vi "cool_amp.vi"() -> ()   [LabVIEW 2011]
uses:
  <vilib>/LabVIEW Interface for Arduino/Type Defs/Digital Pin.ctl
  <vilib>/LabVIEW Interface for Arduino/Type Defs/Pin Mode.ctl
  <vilib>/LabVIEW Interface for Arduino/LabVIEW Interface for Arduino.lvlib
  <vilib>/Analysis/NI_AALBase.lvlib
panel:
  in  "Tab Control":T1(tab)
  in  "save & stop":bool
  out "System Status":bool
  in  "Clear History":bool
  in  "average time":i32=4 min=0 step=1
  in  "Quit Program":bool
  in  "Start":bool
  in  "Stop":bool
  out "T3 Over Limit":bool caption="T3 over limit"
  out "T2 Over Limit":bool caption="T2 over limit"
  out "T1 Over Limit":bool caption="T1 over limit"
  out "Flow Graph":cluster{dbl[], dbl[]}(graph)
  out "flow rate":dbl=4.0 format="%3.1f"
  out "mean flow":dbl=4.0 format="%5.1f"
  out "total cost ($)":dbl=4.0 format="%05.2f"
  out "total flow (L)":dbl=4.0 format="%6.1g"
  out "current flow rate":dbl(slide)=4.0 scale=0.0..20.0
  out "Temp Graph":cluster{dbl[], dbl[]}[](graph)
  out "delta T3":dbl=4.0 format="%6.1g"
  out "delta T2":dbl=4.0 format="%6.1g"
  out "delta T1":dbl=4.0 format="%6.1g"
  out "T3 average":dbl=4.0 format="%6.1f"
  out "T2 average":dbl=4.0 format="%6.1f"
  out "T1 average":dbl=4.0 format="%6.1f"
  out "T3":dbl(slide) scale=-40.0..40.0 scale format="%#_3f"
  out "T2":dbl(slide) scale=-40.0..40.0 scale format="%#_3f"
  out "T1":dbl(slide) scale=-40.0..40.0
  out "T1 numeric":dbl=4.0 format="%6.1f"
  out "T2 numeric":dbl=4.0 format="%6.1f"
  out "T3 numeric":dbl=4.0 format="%6.1f"
  out "T1 max":dbl=4.0 format="%0#3_3g"
  out "T1 min":dbl=4.0 format="%0#3_3g"
  out "T1 average":dbl=4.0 format="%0#3_3g"
  out "T2 max":dbl=4.0 format="%0#3_3g"
  out "T2 min":dbl=4.0 format="%0#3_3g"
  out "T2 average":dbl=4.0 format="%0#3_3g"
  out "T3 max":dbl=4.0 format="%0#3_3g"
  out "T3 min":dbl=4.0 format="%0#3_3g"
  out "T3 average":dbl=4.0 format="%0#3_3g"
  out "max flow":dbl=4.0 format="%#3.1p"
  out "min flow":dbl=4.0 format="%5.1f"
  out "average flow":dbl=4.0 format="%#5.1f"
  out "Arduino \nConnection":bool
  in  "Arduino Serial Port":refnum<visa-resource-name>="ArduinoUno"
  in  "Flow Low Limit":dbl=3.0 min=0.0
  in  "T3 High Limit":dbl=30.0
  in  "T2 High Limit":dbl=30.0
  in  "T1 High Limit":dbl=-20.0
  in  "LED Pin":T2=enum."Pin13"
  out "Total Count":u32=4
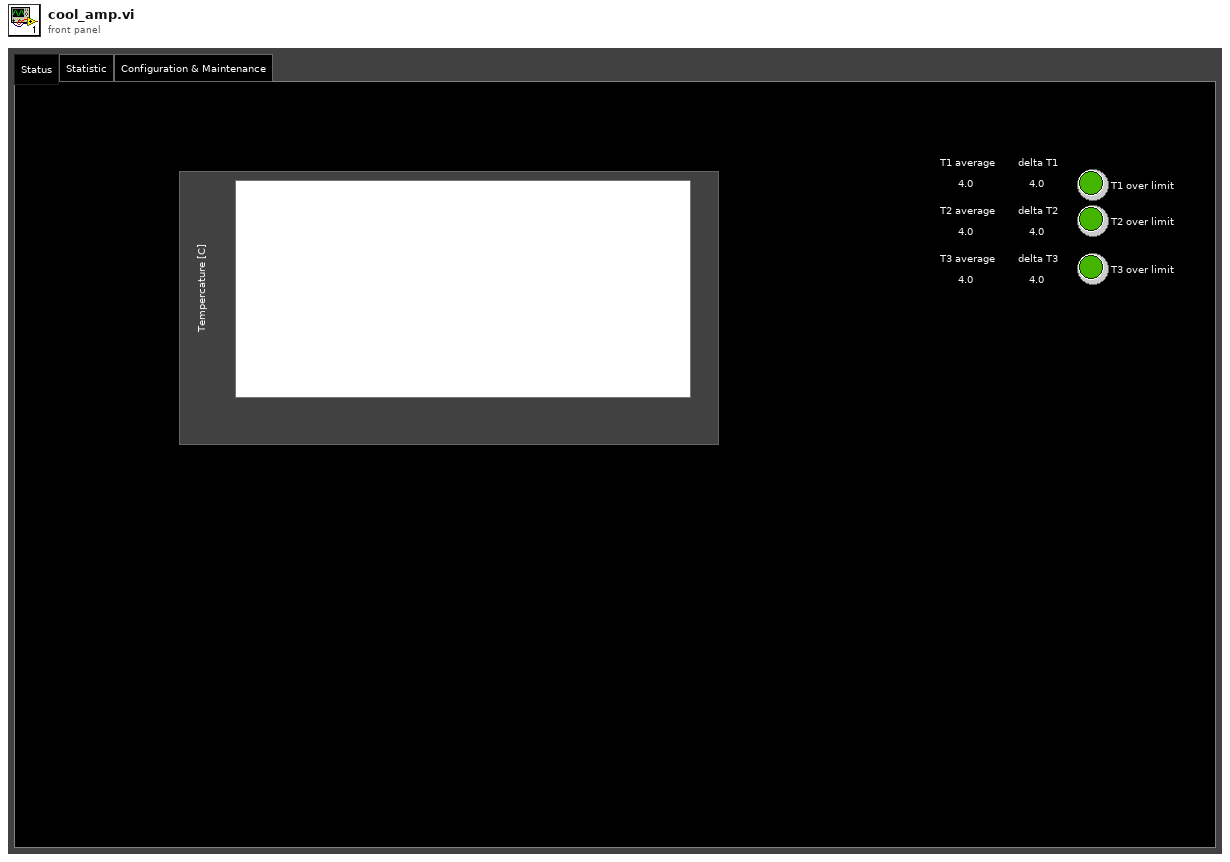
[diagram p1: front panel]
types:
  T1 = enum32{"Status", "Statistic", "Configuration & Maintenance"}
  T2 = typedef "LabVIEW Interface for Arduino.lvlib/Digital Pin.ctl" = enum8{"Pin0", "Pin1", "Pin2", "Pin3", "Pin4", "Pin5", "Pin6", "Pin7", "Pin8", "Pin9", "Pin10", "Pin11", "Pin12", "Pin13"}
  T3 = enum8{"Enabled", "Disabled", "Disabled and Grayed Out"}
  T4 = enum8{"setArduinoMode", "flushSerial", "setPinMode", "digitalWritePin", "digitalWritePort", "tone", "digitalReadPin", "digitalReadPort", "analogReadPin", "analogReadPort", "pwmWritePin", "pwmWritePort", "sevenSegment_Configure", "sevenSegment_Write", "I2C Init", "I2C Write", "I2C Read", "SPI Init", "SPI Set Bit Order", "SPI Set Clock Divider", "SPI Set Data Mode", "SPI Send / Receive", "SPI Close", "Servo Set Num Servos", "Servo Config Servo", "Servo Write Angle", "Servo Read Angle", "Servo Write Pulse Width", "Servo Read Pulse Width", "Servo Detach", "LCD Init", "LCD Set Size", "LCD Set Cursor Mode", "LCD Clear", "LCD Set Cursor Position", "LCD Print", "LCD Display Power", "LCD Scroll Display", "LCD Autoscroll", "LCD Print Direction", "LCD Create Custom Char", "LCD Print Custom Char", "contAcqOn", "contAcqOff", "getFirmwareVersion", "FiniteSampleStart", "readFlowmeter_freq", "readFlowmeter_totalcount"}
  T5 = typedef "LabVIEW Interface for Arduino.lvlib/Pin Mode.ctl" = enum8{"Input", "Output"}
  T6 = typedef "LabVIEW Interface for Arduino.lvlib/Arduino Resource.ctl" = cluster{"VISA resource":refnum<visa-resource-name>, "Board Type":T7, "Connection Type":enum8{"USB / Serial"}, "Bytes Per Packet (15)":u8}
  T7 = typedef "LabVIEW Interface for Arduino.lvlib/Board Type.ctl" = enum16{"Uno", "Dimuelanove w/Atmega 328", "Mega 2560"}
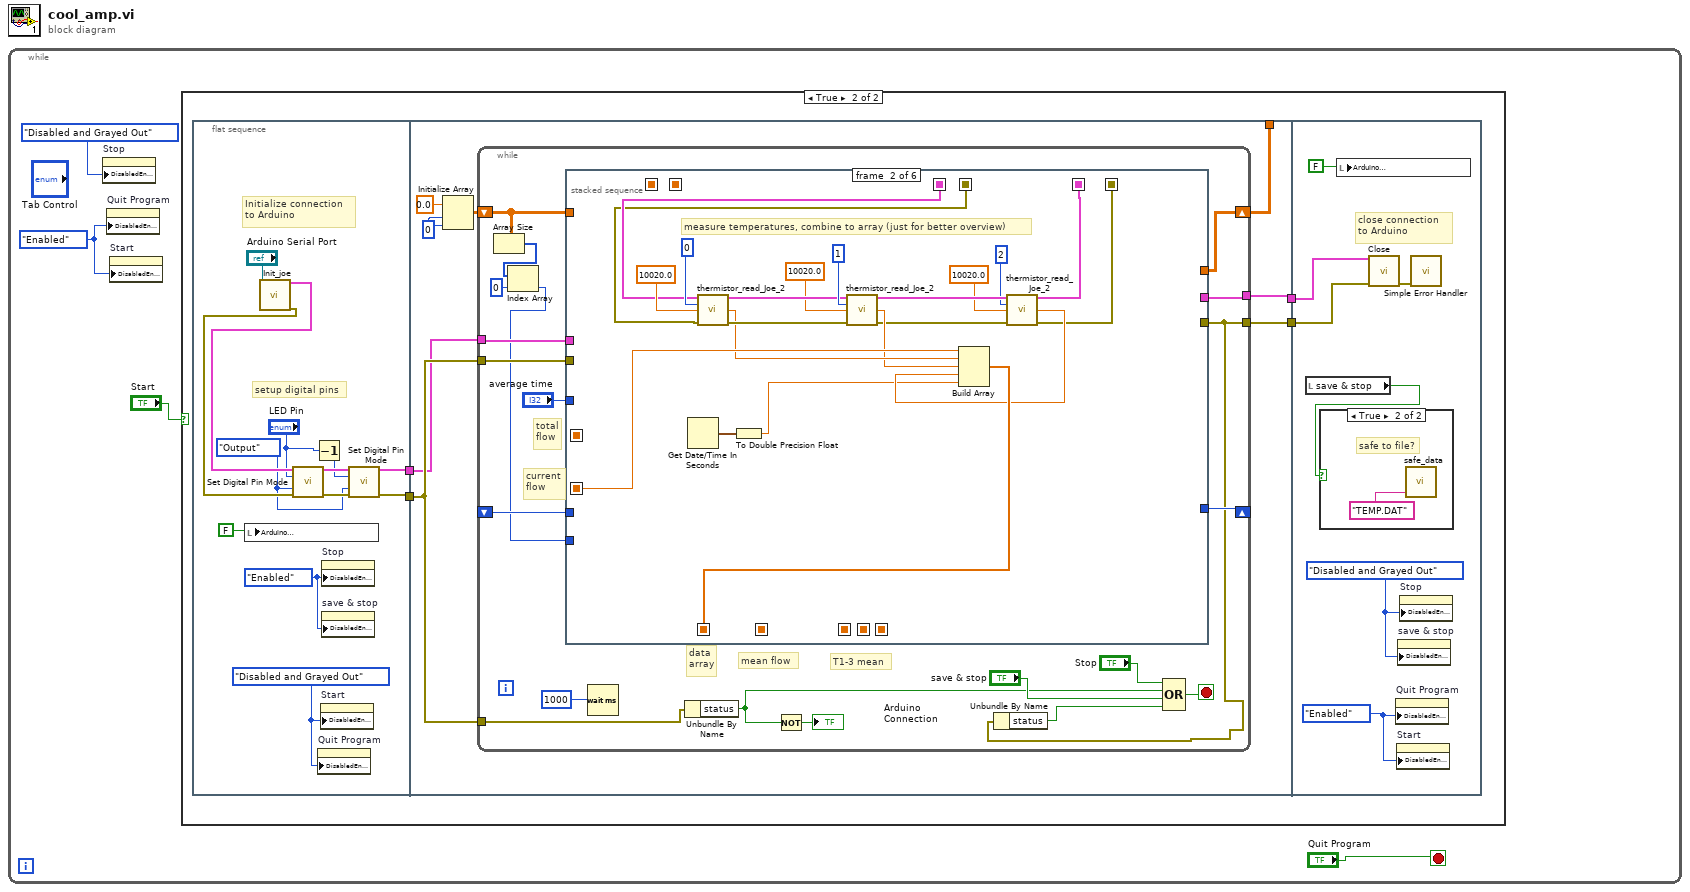
[diagram p0: block diagram]
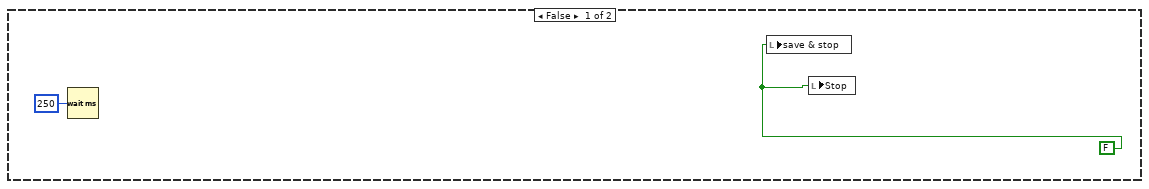
[diagram p2: hidden frame]
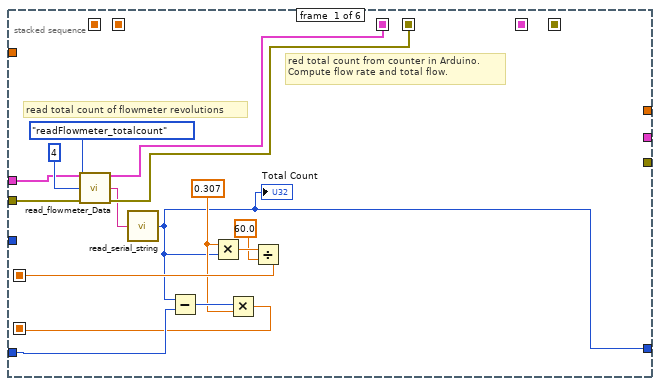
[diagram p3: hidden frame]
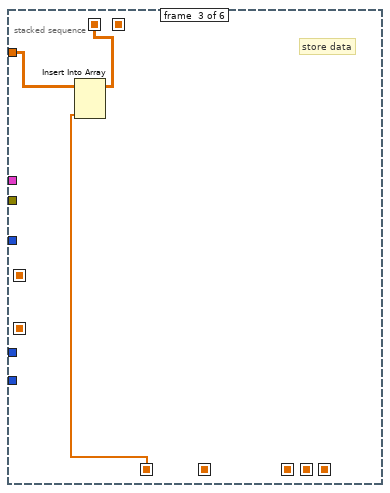
[diagram p4: hidden frame]
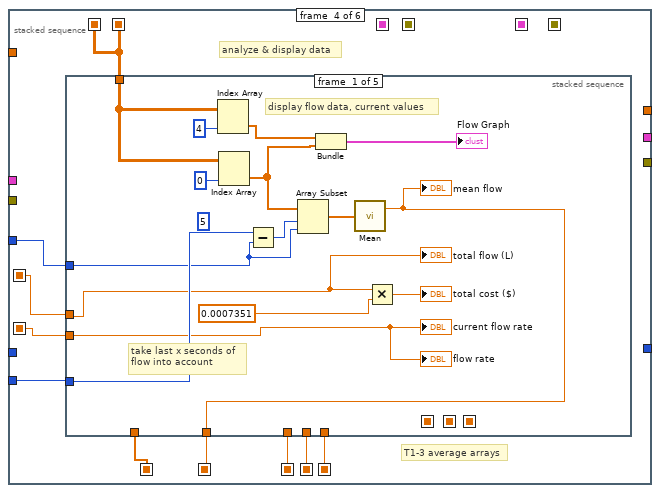
[diagram p5: hidden frame]
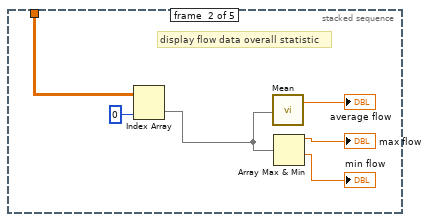
[diagram p6: hidden frame]
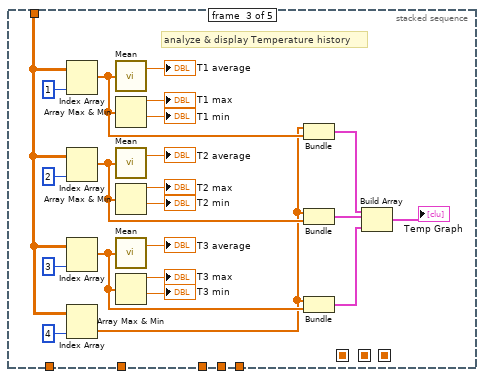
[diagram p7: hidden frame]
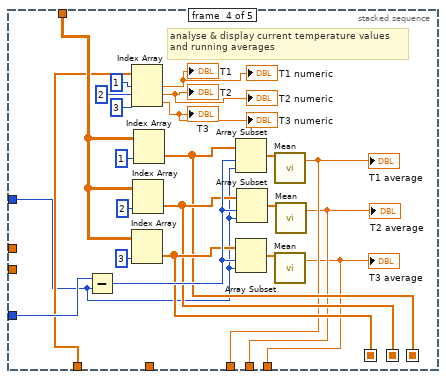
[diagram p8: hidden frame]
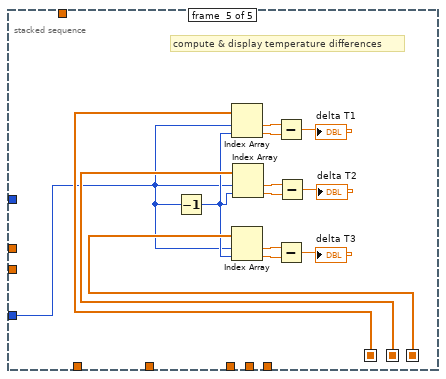
[diagram p9: hidden frame]
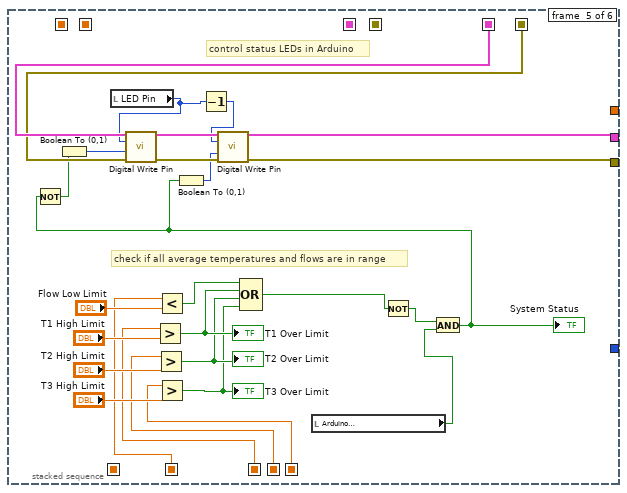
[diagram p10: hidden frame]
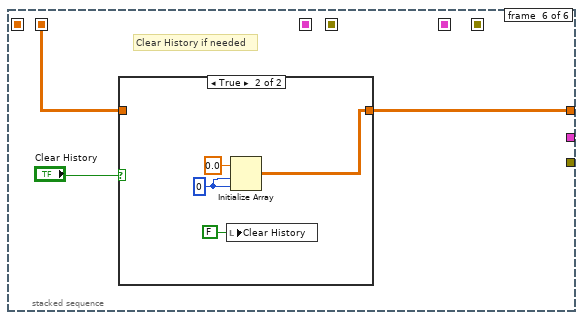
[diagram p11: hidden frame]
diagram:
  n1 = while {
    stop <- "Quit Program" stop-if-true
    w2 = T3."Enabled" ("Disabled")
    n2 = property on="Stop" class="Bool (strict)"("DisabledEnum"=T3."Disabled and Grayed Out" ("Disabled")) -> ()  [unwired: 2 in, 2 out]
    n3 = property on="Quit Program" class="Bool"("DisabledEnum"=w2) -> ()  [unwired: 2 in, 2 out]
    n4 = property on="Start" class="Bool"("DisabledEnum"=w2) -> ()  [unwired: 2 in, 2 out]
    n5 = case shown="True" "Start" {
      frame False {
        w5 = FALSE
        n6 = Wait (ms)(milliseconds to wait=u32 250) -> ()  [unwired: 1 out]
        n7 = local write "save & stop"(w5) -> ()
        n8 = local write "Stop"(w5) -> ()
      }
      frame True {
        n9 = flat-sequence {
          tunnel: [w16] -> w10
          tunnel: [w18] -> w9
          tunnel: w10 -> [w29]
          tunnel: w9 -> [w31]
          tunnel: [w28] -> w8
          tunnel: [w27] -> w7
          tunnel: [w24] -> _
          tunnel: w8 -> [w219]
          tunnel: w7 -> [w220]
          frame #0 {
            w13 = Pin_Mode."Output" ("Pin Mode (Input)")
            w12 = T3."Enabled" ("Disabled")
            w11 = T3."Disabled and Grayed Out" ("Disabled")
            # "setup digital pins"
            # "Initialize connection \nto Arduino"
            n10 = local write "Arduino \nConnection"(FALSE) -> ()
            n11 = call "Init_joe.vi"("VISA resource"="Arduino Serial Port") -> ("Arduino Resource"=w19:T6, "error out"=w21:errorcluster)  [unwired: 17 in]
            n12 = call <vilib>:"Set Digital Pin Mode.vi"("Arduino Resource"=w19, "Digital I/O Pin"="LED Pin", "Pin Mode (Input)"=w13, "error in"=w21) -> ("Arduino Resource"=w17:T6, "error out"=w20:errorcluster)  [unwired: 10 in]
            n13 = Decrement(x="LED Pin") -> (x-1=w14:T2)
            n14 = property on="Quit Program" class="Bool"("DisabledEnum"=w11) -> ()  [unwired: 2 in, 2 out]
            n15 = property on="Start" class="Bool"("DisabledEnum"=w11) -> ()  [unwired: 2 in, 2 out]
            n16 = property on="Stop" class="Bool (strict)"("DisabledEnum"=w12) -> ()  [unwired: 2 in, 2 out]
            n17 = property on="save & stop" class="Bool (strict)"("DisabledEnum"=w12) -> ()  [unwired: 2 in, 2 out]
            n18 = call <vilib>:"Set Digital Pin Mode.vi"("Arduino Resource"=w17, "Digital I/O Pin"=w14, "Pin Mode (Input)"=w13, "error in"=w20) -> ("Arduino Resource"=w16:T6, "error out"=w18:errorcluster)  [unwired: 10 in]
          }
          frame #1 {
            w30 = 0 ("dimension size")
            n19 = Initialize Array(0.0 ("element"), w30, w30) -> (w25:dbl[][])
            n20 = while {
              tunnel: w29 -> [w47]
              tunnel: w31 -> [w46]
              shift-right: [w43] -> w24
              shift-left: w25 -> [w42]
              tunnel: w31 -> [w49]
              tunnel: [w48] -> w28
              tunnel: [w34] -> w27
              shift-right: [w44] -> _
              shift-left: _ -> [w45]
              stop <- w37 stop-if-true
              # "mean flow"
              # "T1-3 mean"
              # "total\nflow"
              # "data\narray"
              # "current\nflow"
              n21 = Array Size(array=w42) -> (size(s)=w41:i32[])
              n22 = Index Array(array=w41, index=0) -> (element=w33:i32)
              n23 = stacked-sequence {
                seq-local: [w52 _ _ _ _ _] -> [_ w81 _ _ _ _]
                seq-local: [w58 _ _ _ _ _] -> [_ w80 _ _ _ _]
                seq-local: [w54 _ _ _ _ _] -> [_ w79 _ w99 _ _]
                seq-local: [_ w77 _ _ _ _] -> [_ _ w88 w93 _ _]
                seq-local: [w62 _ _ _ _ _] -> [_ _ _ w98 _ _]
                seq-local: [_ w70 _ _ _ _] -> [_ _ _ _ w190 _]
                seq-local: [_ w69 _ _ _ _] -> [_ _ _ _ w189 _]
                seq-local: [_ _ _ w91 _ _] -> [_ _ _ _ _ w210]
                seq-local: [_ _ _ w97 _ _] -> [_ _ _ _ w199 _]
                seq-local: [_ _ _ w96 _ _] -> [_ _ _ _ w198 _]
                seq-local: [_ _ _ w95 _ _] -> [_ _ _ _ w197 _]
                seq-local: [_ _ _ w94 _ _] -> [_ _ _ _ w195 _]
                seq-local: [_ _ w89 _ _ _] -> [_ _ _ w91 _ _]
                tunnel: [_ _ _ _ w188 _] -> w48
                tunnel: [_ _ _ _ w186 _] -> w34
                tunnel: w47 -> [w61 _ _ _ _ _]
                tunnel: w46 -> [w60 _ _ _ _ _]
                tunnel: w42 -> [_ _ w90 _ _ _]
                tunnel: w33 -> [_ _ _ w100 _ _]
                tunnel: w45 -> [w56 _ _ _ _ _]
                tunnel: [w53 _ _ _ _ _] -> w44
                tunnel: [_ _ _ _ _ w209] -> w43
                tunnel: "average time" -> [_ _ _ w92 _ _]
                frame #0 {
                  w55 = 0.307
                  # "read total count of flowmeter revolutions"
                  # "red total count from counter in Arduino. \nCompute flow rate and total flow."
                  n24 = call "read_flowmeter_Data.vi"("Arduino Resource"=w61, "Command"=T4."readFlowmeter_totalcount", "Bytes To Read (0)"=u8 4, "error in"=w60) -> ("Arduino Resource"=w52:T6, "Read Buffer"=w57:string, "error out"=w58:errorcluster)  [unwired: 9 in]
                  n25 = call "read_serial_string.vi"("serial read Buffer"=w57) -> ("unsigned long"=w53:u32)  [unwired: 4 in]
                  "Total Count" <- w53
                  n26 = Subtract(x=w53, y=w56) -> (x-y=w59:u32)
                  n27 = Multiply(x=w55, y=w53) -> (x*y=w64:dbl)
                  n28 = Multiply(x=w59, y=w55) -> (x*y=w54:dbl)
                  n29 = Divide(x=w64, y=60.0) -> (x/y=w62:dbl)
                }
                frame #1 {
                  # "measure temperatures, combine to array (just for better overview)"
                  n30 = Get Date/Time In Seconds() -> (seconds since 1Jan1904=w68:timestamp)
                  n31 = call "thermistor_read_Joe_2.vi"("Arduino Resource"=w81, "Thermistor AI Pin (0)"=u8 0 ("T1 Pin"), "Paired Resistance (10K Ohms)"=10020.0, "error in"=w80) -> ("Arduino Resource"=w84:T6, "Temperature"=w78:dbl, "error out"=w83:errorcluster)  [unwired: 9 in]
                  n32 = To Double Precision Float(number=w68) -> (double precision float=w67:dbl)
                  n33 = call "thermistor_read_Joe_2.vi"("Arduino Resource"=w84, "Thermistor AI Pin (0)"=u8 1 ("T2 Pin"), "Paired Resistance (10K Ohms)"=10020.0, "error in"=w83) -> ("Arduino Resource"=w75:T6, "Temperature"=w76:dbl, "error out"=w74:errorcluster)  [unwired: 9 in]
                  n34 = call "thermistor_read_Joe_2.vi"("Arduino Resource"=w75, "Thermistor AI Pin (0)"=u8 2 ("T2 Pin"), "Paired Resistance (10K Ohms)"=10020.0, "error in"=w74) -> ("Arduino Resource"=w70:T6, "Temperature"=w71:dbl, "error out"=w69:errorcluster)  [unwired: 9 in]
                  n35 = Build Array(w79, w78, w76, w71, w67) -> (w77:dbl[])
                }
                frame #2 {
                  # "store data"
                  n36 = Insert Into Array(array=w90, new element=w88) -> (w89:dbl[][])  [unwired: 2 in]
                }
                frame #3 {
                  # "T1-3 average arrays"
                  # "analyze & display data"
                  n37 = stacked-sequence {
                    seq-local: [_ _ _ w151 _] -> [_ _ _ _ w180]
                    seq-local: [_ _ _ w150 _] -> [_ _ _ _ w170]
                    seq-local: [_ _ _ w148 _] -> [_ _ _ _ w169]
                    tunnel: w91 -> [w102 w117 w124 w159 _]
                    tunnel: w100 -> [w113 _ _ w162 w167]
                    tunnel: w99 -> [w108 _ _ _ _]
                    tunnel: w98 -> [w109 _ _ _ _]
                    tunnel: w93 -> [_ _ _ w149 _]
                    tunnel: [_ _ _ w147 _] -> w97
                    tunnel: [_ _ _ w146 _] -> w96
                    tunnel: [_ _ _ w145 _] -> w95
                    tunnel: [w105 _ _ _ _] -> w94
                    tunnel: w92 -> [w104 _ _ w144 _]
                    frame #0 {
                      (unwired) 5 ("disabled index (col)")
                      # "display flow data, current values"
                      # "take last x seconds of \nflow into account"
                      n38 = Index Array(array=w102, index (col)=4 ("disabled index (col)")) -> (element=w103:dbl[])  [unwired: 1 in]
                      n39 = Index Array(array=w102, index (col)=0 ("disabled index (col)")) -> (element=w106:dbl[])  [unwired: 1 in]
                      n40 = Subtract(x=w113, y=w104) -> (x-y=w114:i32)
                      n41 = Array Subset(array=w106, index=w114, length=w104) -> (w112:dbl[])
                      n42 = Bundle(w103, w106) -> (→"Flow Graph":cluster{dbl[], dbl[]})  [unwired: 1 in]
                      n43 = call <vilib>:"Mean.vi"("X"=w112) -> ("mean"=w105:dbl)  [unwired: 1 out]
                      "mean flow" <- w105
                      n44 = Multiply(x=w109, y=0.0007351) -> (x*y=→"total cost ($)":dbl)
                      "current flow rate" <- w108
                      "total flow (L)" <- w109
                      "flow rate" <- w108
                    }
                    frame #1 {
                      # "display flow data overall statistic"
                      n45 = Index Array(array=w117, index (col)=0 ("disabled index (col)")) -> (element=w116:dbl[])  [unwired: 1 in]
                      n46 = call <vilib>:"Mean.vi"("X"=w116) -> ("mean"=→"average flow":dbl)  [unwired: 1 out]
                      n47 = Array Max & Min(array=w116) -> (max value=→"max flow":dbl, min value=→"min flow":dbl)  [unwired: 2 out]
                    }
                    frame #2 {
                      # "analyze & display Temperature history"
                      n48 = Index Array(array=w124, index (col)=1 ("disabled index (col)")) -> (element=w128:dbl[])  [unwired: 1 in]
                      n49 = Index Array(array=w124, index (col)=2 ("disabled index (col)")) -> (element=w127:dbl[])  [unwired: 1 in]
                      n50 = Index Array(array=w124, index (col)=3 ("disabled index (col)")) -> (element=w126:dbl[])  [unwired: 1 in]
                      n51 = Index Array(array=w124, index (col)=4 ("disabled index (col)")) -> (element=w123:dbl[])  [unwired: 1 in]
                      n52 = call <vilib>:"Mean.vi"("X"=w128) -> ("mean"=→"T1 average":dbl)  [unwired: 1 out]
                      n53 = Array Max & Min(array=w128) -> (max value=→"T1 max":dbl, min value=→"T1 min":dbl)  [unwired: 2 out]
                      n54 = call <vilib>:"Mean.vi"("X"=w127) -> ("mean"=→"T2 average":dbl)  [unwired: 1 out]
                      n55 = Array Max & Min(array=w127) -> (max value=→"T2 max":dbl, min value=→"T2 min":dbl)  [unwired: 2 out]
                      n56 = call <vilib>:"Mean.vi"("X"=w126) -> ("mean"=→"T3 average":dbl)  [unwired: 1 out]
                      n57 = Array Max & Min(array=w126) -> (max value=→"T3 max":dbl, min value=→"T3 min":dbl)  [unwired: 2 out]
                      n58 = Bundle(w123, w128) -> (w130:cluster{dbl[], dbl[]})  [unwired: 1 in]
                      n59 = Bundle(w123, w127) -> (w131:cluster{dbl[], dbl[]})  [unwired: 1 in]
                      n60 = Bundle(w123, w126) -> (w129:cluster{dbl[], dbl[]})  [unwired: 1 in]
                      n61 = Build Array(w130, w131, w129) -> (→"Temp Graph":cluster{dbl[], dbl[]}[])
                    }
                    frame #3 {
                      # "analyse & display current temperature values\nand running averages"
                      n62 = Subtract(x=w162, y=w144) -> (x-y=w158:i32)
                      n63 = Index Array(array=w149, index #1=1, index #2=2, index #3=3) -> (element #1=→"T1" →"T1 numeric":dbl, element #2=→"T2" →"T2 numeric":dbl, element #3=→"T3" →"T3 numeric":dbl)
                      n64 = Index Array(array=w159, index (col)=3 ("disabled index (col)")) -> (element=w151:dbl[])  [unwired: 1 in]
                      n65 = Index Array(array=w159, index (col)=2 ("disabled index (col)")) -> (element=w150:dbl[])  [unwired: 1 in]
                      n66 = Index Array(array=w159, index (col)=1 ("disabled index (col)")) -> (element=w148:dbl[])  [unwired: 1 in]
                      n67 = Array Subset(array=w148, index=w158, length=w144) -> (w153:dbl[])
                      n68 = Array Subset(array=w151, index=w158, length=w144) -> (w154:dbl[])
                      n69 = Array Subset(array=w150, index=w158, length=w144) -> (w152:dbl[])
                      n70 = call <vilib>:"Mean.vi"("X"=w153) -> ("mean"=w147:dbl)  [unwired: 1 out]
                      "T1 average" <- w147
                      n71 = call <vilib>:"Mean.vi"("X"=w154) -> ("mean"=w145:dbl)  [unwired: 1 out]
                      "T3 average" <- w145
                      n72 = call <vilib>:"Mean.vi"("X"=w152) -> ("mean"=w146:dbl)  [unwired: 1 out]
                      "T2 average" <- w146
                    }
                    frame #4 {
                      # "compute & display temperature differences"
                      n73 = Decrement(x=w167) -> (x-1=w168:i32)
                      n74 = Index Array(array=w180, index #1=w167, index #2=w168) -> (element #1=w179:dbl, element #2=w178:dbl)
                      n75 = Index Array(array=w169, index #1=w167, index #2=w168) -> (element #1=w173:dbl, element #2=w172:dbl)
                      n76 = Index Array(array=w170, index #1=w167, index #2=w168) -> (element #1=w176:dbl, element #2=w175:dbl)
                      n77 = Subtract(x=w179, y=w178) -> (x-y=→"delta T1":dbl)
                      n78 = Subtract(x=w173, y=w172) -> (x-y=→"delta T3":dbl)
                      n79 = Subtract(x=w176, y=w175) -> (x-y=→"delta T2":dbl)
                    }
                  }
                }
                frame #4 {
                  # "check if all average temperatures and flows are in range"
                  # "control status LEDs in Arduino"
                  n80 = local read "LED Pin"() -> (w185:T2)
                  n81 = Greater?(x=w199, y="T1 High Limit") -> (0:w203:bool)
                  "T1 Over Limit" <- w203
                  n82 = Greater?(x=w198, y="T2 High Limit") -> (0:w202:bool)
                  "T2 Over Limit" <- w202
                  n83 = Less?(x=w195, y="Flow Low Limit") -> (x < y?=w194:bool)
                  n84 = Greater?(x=w197, y="T3 High Limit") -> (0:w201:bool)
                  "T3 Over Limit" <- w201
                  n85 = Decrement(x=w185) -> (x-1=w184:T2)
                  n86 = Compound Arithmetic op=OR(w194, w203, w202, w201) -> (w192:bool)
                  n87 = local read "Arduino \nConnection"() -> (w193:bool)
                  n88 = Not(x=w192) -> (.not. x?=w191:bool)
                  n89 = And(x=w191, y=w193) -> (x .and. y?=w182:bool)
                  "System Status" <- w182
                  n90 = Not(x=w182) -> (.not. x?=w181:bool)
                  n91 = Boolean To (0,1)(Boolean=w181) -> (0, 1=w200:i16)
                  n92 = call <vilib>:"Digital Write Pin.vi"("Arduino Resource"=w190, "Digital I/O Pin (0)"=w185, "Value (0)"=w200, "error in"=w189) -> ("Arduino Resource"=w207:T6, "error out"=w187:errorcluster)  [unwired: 10 in]
                  n93 = Boolean To (0,1)(Boolean=w182) -> (0, 1=w183:i16)
                  n94 = call <vilib>:"Digital Write Pin.vi"("Arduino Resource"=w207, "Digital I/O Pin (0)"=w184, "Value (0)"=w183, "error in"=w187) -> ("Arduino Resource"=w188:T6, "error out"=w186:errorcluster)  [unwired: 10 in]
                }
                frame #5 {
                  # "Clear History if needed"
                  n95 = case shown="True" "Clear History" {
                    tunnel: w210 -> [w211 _]
                    tunnel: [w211 w213] -> w209
                    frame False {
                    }
                    frame True {
                      w215 = 0 ("dimension size")
                      n96 = local write "Clear History"(FALSE ("Clear History")) -> ()
                      n97 = Initialize Array(0.0 ("element"), w215, w215) -> (w213:dbl[][])
                    }
                  }
                }
              }
              n98 = Wait (ms)(milliseconds to wait=u32 1000) -> ()  [unwired: 1 out]
              n99 = Unbundle By Name(w49) -> ("status"=w36:bool)
              n100 = Not(x=w36) -> (.not. x?=→"Arduino \nConnection":bool)
              n101 = Unbundle By Name(w34) -> ("status"=w35:bool)
              n102 = Compound Arithmetic op=OR("Stop", w36, "save & stop", w35) -> (w37:bool)
            }
          }
          frame #2 {
            w217 = T3."Disabled and Grayed Out" ("Disabled")
            w218 = T3."Enabled" ("Disabled")
            # "close connection \nto Arduino"
            n103 = local read "save & stop"() -> (w216:bool)
            n104 = case shown="True" w216 {
              frame False {
              }
              frame True {
                # "safe to file?"
                n105 = call "safe_data.vi"("default name"="TEMP.DAT") -> ()  [unwired: 6 in]
              }
            }
            n106 = local write "Arduino \nConnection"(FALSE) -> ()
            n107 = call <vilib>:"Close.vi"("Arduino Resource"=w219, "error in"=w220) -> ("error out"=w222:errorcluster)  [unwired: 13 in]
            n108 = property on="Quit Program" class="Bool"("DisabledEnum"=w218) -> ()  [unwired: 2 in, 2 out]
            n109 = property on="Start" class="Bool"("DisabledEnum"=w218) -> ()  [unwired: 2 in, 2 out]
            n110 = property on="save & stop" class="Bool (strict)"("DisabledEnum"=w217) -> ()  [unwired: 2 in, 2 out]
            n111 = property on="Stop" class="Bool (strict)"("DisabledEnum"=w217) -> ()  [unwired: 2 in, 2 out]
            n112 = call <vilib>:"Simple Error Handler.vi"("error in (no error)"=w222) -> ()  [unwired: 4 in, 5 out]
          }
        }
      }
    }
  }
